vi "Read Meter.vi"(8 "error in (no error)":errorcluster, 11 "OD600 in":refnum<class "OD600.lvclass">) -> (0 "error out":errorcluster, 3 "OD600 out":refnum<class "OD600.lvclass">)   [LabVIEW 2013, in "OD600.lvlib" / "OD600.lvclass"]
uses:
  OD600.lvclass
  OD600.lvclass/OD600.ctl
  <vilib>/Analysis/6fits.llb/Curve Fitting Criteria.ctl
  Read VISA 1.vi
  Read Window Size.vi
  Read OD600.vi
  Read Growth Rate.vi
  PluginInterface/PluginInterface.lvlibp/PluginInterfaceClass/Read DVR.vi
  PluginInterface/PluginInterface.lvlibp/PluginInterfaceClass/Read TDMS.vi
  PluginInterface/PluginInterface.lvlibp/PluginInterfaceClass/Read Name.vi
  <vilib>/Analysis/NI_AALPro.lvlib
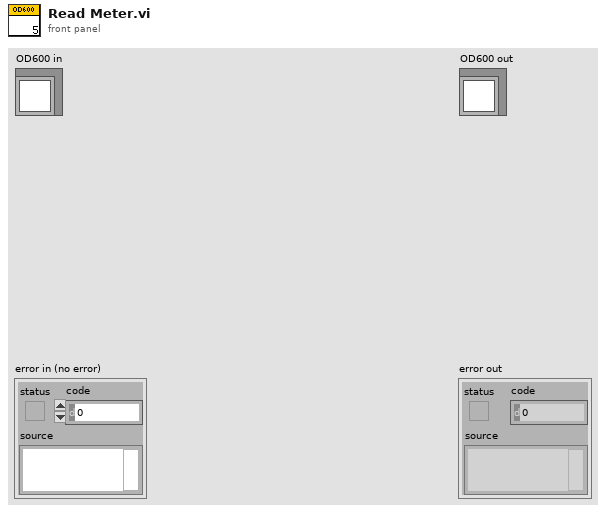
[diagram p1: front panel]
types:
  T1 = typedef "NI_AALPro.lvlib/Curve Fitting Criteria.ctl" = u16
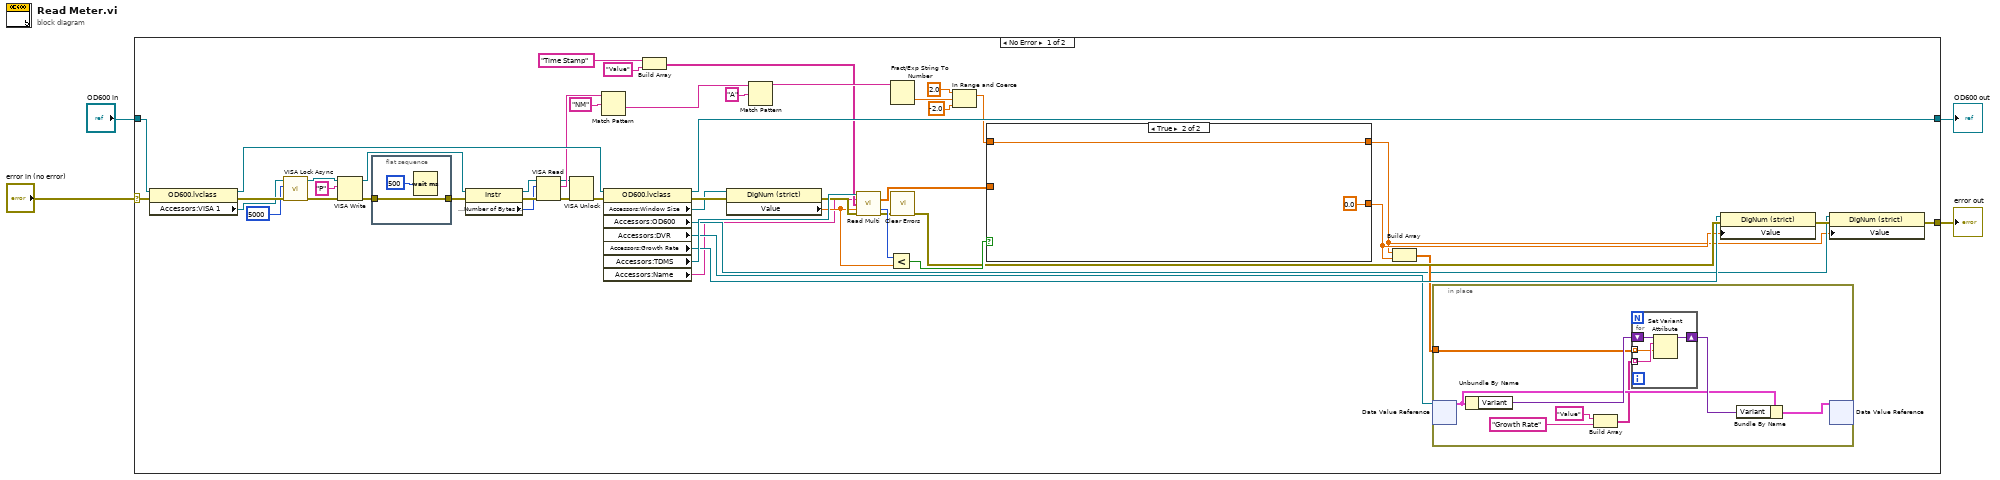
[diagram p0: block diagram]
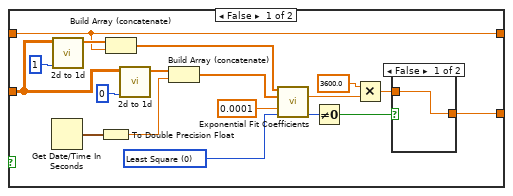
[diagram p2: hidden frame]
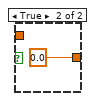
[diagram p3: hidden frame]
diagram:
  n1 = case shown="No Error" "error in (no error)" {
    selector: "error in (no error)" -> [w53 w92]
    tunnel: [w6 w92] -> w1
    tunnel: [w36 w91] -> w2
    tunnel: "OD600 in" -> [w54 w91]
    frame No Error {
      n2 = property class="OD600.lvclass"(reference=w54, error in=w53) -> (reference out=w50:refnum<class "OD600.lvclass">, error out=w16:errorcluster, "Accessors:VISA 1"=w14:refnum<visa-resource-name>)
      n3 = call <vilib>:"VISA Lock Async.vi"("error in (no error)"=w16, "timeout (0)"=u32 5000, "VISA resource name"=w14) -> ("error out"=w15:errorcluster, "VISA resource name out"=w13:refnum<visa-resource-name>)  [unwired: 6 in, 1 out]
      n4 = VISA Write(VISA resource name=w13, write buffer="P" ("string"), error in (no error)=w15) -> (VISA resource name out=w46:refnum<visa-resource-name>, error out=w52:errorcluster)  [unwired: 1 out]
      n5 = flat-sequence {
        tunnel: [w89] -> w49
        tunnel: w52 -> [w89]
        frame #0 {
          n6 = Wait (ms)(milliseconds to wait=u32 500) -> ()  [unwired: 1 out]
        }
      }
      n7 = property class="Instr"(reference=w46, error in=w49) -> (reference out=w45:refnum<visa-resource-name>, error out=w48:errorcluster, "Serial Settings:Number of Bytes at Serial Port"=w47:u32)
      n8 = VISA Read(VISA resource name=w45, byte count=w47, error in (no error)=w48) -> (VISA resource name out=w11:refnum<visa-resource-name>, read buffer=w44:string, error out=w10:errorcluster)  [unwired: 1 out]
      n9 = VISA Unlock(8:w10, 11:w11) -> (0:w9:errorcluster)  [unwired: 1 out]
      n10 = Match Pattern(string=w44, regular expression="NM") -> (after substring=w42:string)  [unwired: 1 in, 3 out]
      n11 = property class="OD600.lvclass"(reference=w50, error in=w9) -> (reference out=w36:refnum<class "OD600.lvclass">, error out=w35:errorcluster, "Accessors:Window Size"=w17:refnum<vi>, "Accessors:OD600"=w18:refnum<vi>, "Accessors:DVR"=w21:refnum<data-value>, "Accessors:Growth Rate"=w22:refnum<vi>, "Accessors:TDMS"=w33:refnum<k34>, "Accessors:Name"=w5:string)
      n12 = Build Array("Time Stamp" ("Channel"), "Value" ("string")) -> (w31:string[])
      n13 = property class="DigNum (strict)"(reference=w17, error in=w35) -> (error out=w24:errorcluster, "Value"=w23:dbl)  [unwired: 1 out]
      n14 = Match Pattern(string=w42, regular expression="A") -> (before substring=w40:string)  [unwired: 1 in, 3 out]
      n15 = call "Read Multi.vi"("tdms file in"=w33, "group"=w5, "Channel"=w31, "Numeric"=w23, "error in (no error)"=w24) -> ("Array"=w32:dbl[][], "Length"=w28:u64, "error out"=w26:errorcluster)  [unwired: 7 in, 1 out]
      n16 = Less?(x=w28, y=w23) -> (x < y?=w27:bool)
      n17 = Fract/Exp String To Number(string=w40) -> (number=w39:dbl)  [unwired: 3 in, 1 out]
      n18 = call <vilib>:"Clear Errors.vi"("error in (no error)"=w26) -> ("error out"=w25:errorcluster)  [unwired: 6 in]
      n19 = In Range and Coerce(upper limit=2.0, x=w39, lower limit=-2.0) -> (coerced(x)=w8:dbl)  [unwired: 1 out]
      n20 = case shown="True" w27 {
        tunnel: w32 -> [w84 _]
        tunnel: [w74 0.0 ("damping")] -> w20
        tunnel: w8 -> [w67 w87]
        tunnel: [w67 w87] -> w7
        frame False {
          w81 = T1 0 items=["Least Square", "Least Absolute Residual", "Bisquare"] ("method")
          n21 = Get Date/Time In Seconds() -> (seconds since 1Jan1904=w71:timestamp)
          n22 = call "2d to 1d.vi"("index"=1, "array"=w84) -> ("output array"=w73:dbl[])  [unwired: 9 in]
          n23 = To Double Precision Float(number=w71) -> (double precision float=w70:dbl)
          n24 = Build Array (concatenate)(w73, w67) -> (w69:dbl[])
          n25 = call "2d to 1d.vi"("index"=0, "array"=w84) -> ("output array"=w72:dbl[])  [unwired: 9 in]
          n26 = Build Array (concatenate)(w72, w70) -> (w68:dbl[])
          n27 = call <vilib>:"Exponential Fit Coefficients.vi"("Y"=w69, "X"=w68, "tolerance"=0.0001, "method"=w81) -> ("damping"=w77:dbl, "error"=w79:i32)  [unwired: 9 in, 1 out]
          n28 = Not Equal To 0?(x=w79) -> (x != 0?=w78:bool)
          n29 = Multiply(x=3600.0, y=w77) -> (x*y=w76:dbl)
          n30 = case shown="False" w78 {
            tunnel: [w85 0.0 ("damping")] -> w74
            tunnel: w76 -> [w85 _]
            frame False {
            }
            frame True {
            }
          }
        }
        frame True {
        }
      }
      n31 = Build Array(w7, w20) -> (w19:dbl[])
      n32 = in-place {
        in-place-border: w19 -> [w55]
        n33 = in-place-dvr #1(w21) -> (w59:cluster{"Array":string[], "Variant":variant})  [unwired: 1 out]
        n34 = Unbundle By Name(w59) -> ("Variant"=w61:variant)
        n35 = Build Array("Value" ("string"), "Growth Rate" ("string")) -> (w56:string[])
        n36 = for {
          tunnel: w56 -> [w64] mode=indexing
          tunnel: w55 -> [w63] mode=indexing
          shift-right: [w65] -> w60
          shift-left: w61 -> [w66]
          n37 = Set Variant Attribute(Variant=w66, name=w64, value=w63) -> (Variant out=w65:variant)  [unwired: 1 in, 2 out]
        }
        n38 = Bundle By Name(cluster=w59, "Variant"=w60) -> (w62:cluster{"Array":string[], "Variant":variant})
        n39 = in-place-dvr #1(w62) -> ()  [unwired: 2 out]
      }
      n40 = property class="DigNum (strict)"(reference=w22, error in=w25, "Value"=w20) -> (error out=w34:errorcluster)  [unwired: 1 out]
      n41 = property class="DigNum (strict)"(reference=w18, error in=w34, "Value"=w7) -> (error out=w6:errorcluster)  [unwired: 1 out]
    }
    frame Error {
    }
  }
  "error out" <- w1
  "OD600 out" <- w2
